vi "Set Position History.vi"(8 "Error In":errorcluster, 10 "Positions History":T1[](array[typedef]), 11 "Pixel In":refnum<class "Pixel.lvclass">) -> (0 "Error Out":errorcluster, 3 "Pixel Out":refnum<class "Pixel.lvclass">)   [LabVIEW 2019, in "Pixel.lvclass"]
uses:
  Pixel.lvclass
  Display Utilities/Public/Controls/2D Coordinates.ctl
  Display Utilities/Display Utilities.lvlib
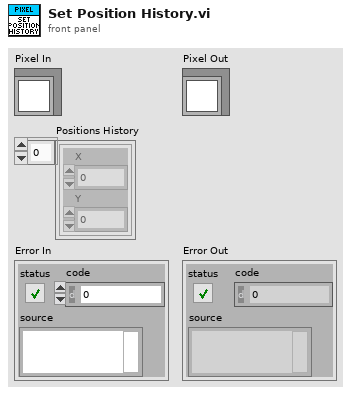
[diagram p1: front panel]
types:
  T1 = typedef "Display Utilities.lvlib/2D Coordinates.ctl" = cluster{"X":i32, "Y":i32}
  T2 = typedef "Pixel.lvclass/Data.ctl" = cluster{"Trace":i32, "Positions History":T3[]}
  T3 = typedef "Display Element.lvclass/Vector.ctl" = cluster{"X":i32, "Y":i32}
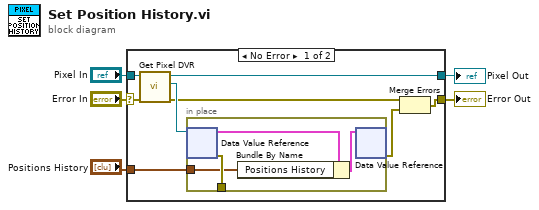
[diagram p0: block diagram]
diagram:
  n1 = case shown="No Error" "Error In" {
    selector: "Error In" -> [w9 w18]
    tunnel: [w12 w18] -> w4
    tunnel: [w7 w19] -> w2
    tunnel: "Pixel In" -> [w10 w19]
    tunnel: "Positions History" -> [w11 _]
    frame No Error {
      n2 = call "Get Pixel DVR.vi"("Error In"=w9, "Pixel In"=w10) -> ("Error Out"=w6:errorcluster, "DVR"=w8:refnum<data-value>, "Pixel Out"=w7:refnum<class "Pixel.lvclass">)  [unwired: 7 in]
      n3 = in-place {
        in-place-border: [w17] -> _
        in-place-border: w11 -> [w14]
        n4 = in-place-dvr #1(w8) -> (w16:T2, w17:errorcluster)
        n5 = Bundle By Name(cluster=w16, "Positions History"=w14) -> (w15:T2)
        n6 = in-place-dvr #1(w15) -> (w13:errorcluster)  [unwired: 1 out]
      }
      n7 = Merge Errors(w6, w13) -> (w12:errorcluster)
    }
    frame Error {
    }
  }
  "Pixel Out" <- w2
  "Error Out" <- w4
